vi "TCP-IP Mgr.Destroy.vi"(8 "error in (no error)":errorcluster, 11 "Q Name":string="TCP-IP Mgr") -> (0 "error out":errorcluster)   [LabVIEW 2024, in "EQMF.lvlib" / "TCP-IP.lvlib"]
uses:
  TCP-IP.lvlib
  Queues/Q.Element.ctl
  Queues/Queue Utils.lvlib
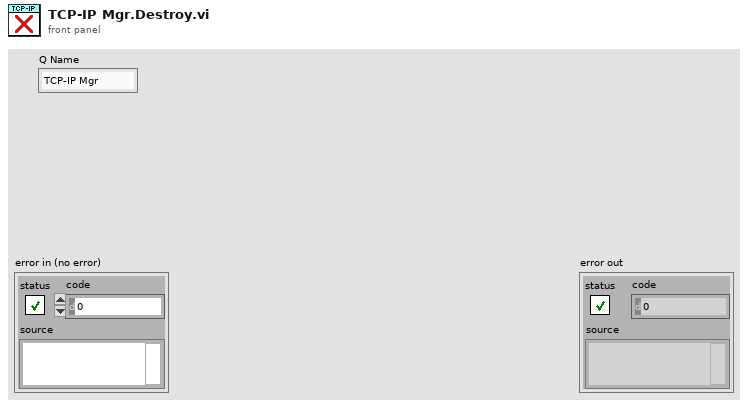
[diagram p1: front panel]
types:
  T1 = typedef "EQMF.lvlib/Queue Utils.lvlib/Q.Element.ctl" = cluster{"Cmd":string, "Sub":string, "Data1":variant, "Data2":variant}
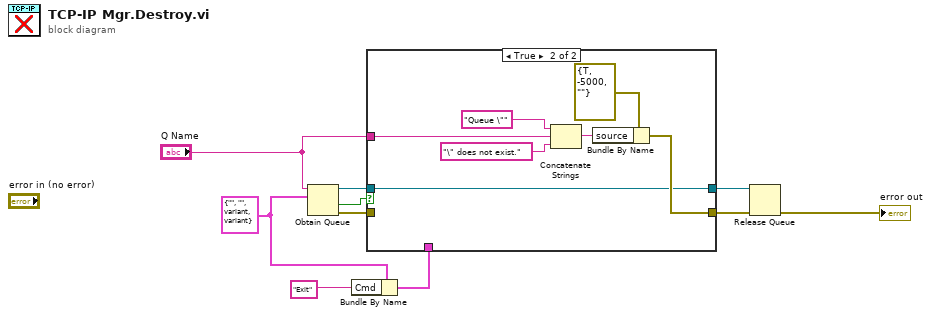
[diagram p0: block diagram]
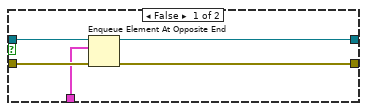
[diagram p2: hidden frame]
diagram:
  w2 = T1 {"Cmd"="", "Sub"="", "Data1"=variant, "Data2"=variant} ("Queue Element")
  n1 = Obtain Queue(name (unnamed)="Q Name", element data type=w2) -> (queue out=w9:refnum<queue>, created new?=w8:bool, error out=w10:errorcluster)  [unwired: 3 in]
  n2 = Bundle By Name(cluster=w2, "Cmd"="Exit") -> (w6:T1)
  n3 = case shown="True" w8 {
    tunnel: w10 -> [w14 _]
    tunnel: w9 -> [w15 w16]
    tunnel: [w11 w18] -> w5
    tunnel: "Q Name" -> [_ w17]
    tunnel: w6 -> [w13 _]
    tunnel: [w12 w16] -> w4
    frame False {
      n4 = Enqueue Element At Opposite End(queue=w15, element=w13, error in (no error)=w14) -> (queue out=w12:refnum<queue>, error out=w11:errorcluster)  [unwired: 1 in, 1 out]
    }
    frame True {
      n5 = Concatenate Strings("Queue \"", w17, "\" does not exist.") -> (w19:string)
      n6 = Bundle By Name(cluster=errorcluster {"status"=TRUE, "code"=-5000, "source"=""} ("error constant"), "source"=w19) -> (w18:errorcluster)
    }
  }
  n7 = Release Queue(queue=w4, error in (no error)=w5) -> (error out=→"error out":errorcluster)  [unwired: 1 in, 2 out]
